vi "ELVIS III v1.1 Open UART.vi"(8 "error in (no error)":errorcluster, 10 "VISA resource name in":refnum<visa-resource-name>, 11 "Resource name":T1 caption="RIO Device") -> (0 "error out":errorcluster, 3 "VISA resource name":refnum<visa-resource-name>)   [LabVIEW 2021]
uses:
  <vilib>/userDefined/High Color/nirio_resource_hc.ctl
  <vilib>/myRIO/Common/Instrument Driver Framework/ELVIS III v1.0/UART/vis/ELVIS III v1.0 Build MUX Configuration UART.vi
  <vilib>/myRIO/Common/Instrument Driver Framework/ELVIS III v1.0/Resource Manager/vis/ELVIS III v1.0 Reserve Channel List.vi
  <vilib>/myRIO/Common/Instrument Driver Framework/ELVIS III v1.0/UART/vis/ELVIS III v1.0 Configure UART.vi
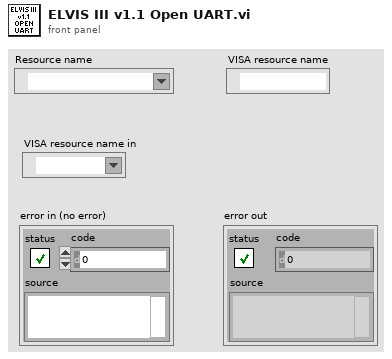
[diagram p1: front panel]
types:
  T1 = typedef "nirio_resource_hc.ctl" = tag
  T2 = typedef "Generic FPGA Reference.ctl" = refnum<k20>
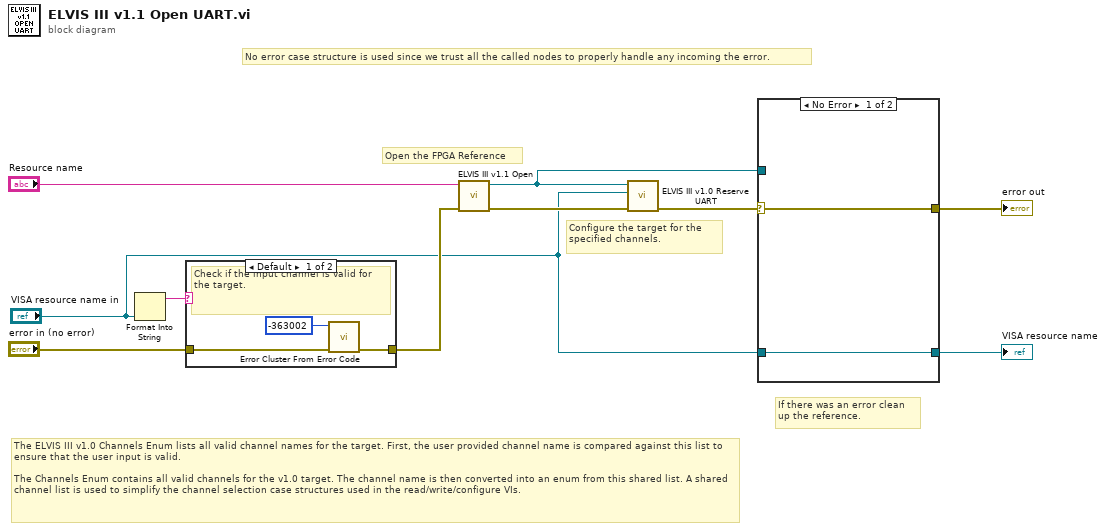
[diagram p0: block diagram]
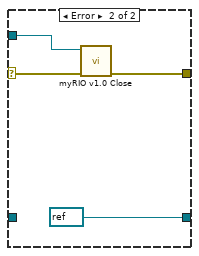
[diagram p3: hidden frame]
diagram:
  # "The ELVIS III v1.0 Channels Enum lists all valid channel names for the target. First, the user provided channel name is compared against this list to ensure that the user input is valid.\n\nThe Channels Enum contains all valid channels for the v1.0 target. The channel name is then converted into an enum from this shared list. A shared channel list is used to simplify the channel selection case structures used in the read/write/configure VIs."
  # "If there was an error clean up the reference."
  # "Configure the target for the specified channels."
  # "Open the FPGA Reference"
  # "No error case structure is used since we trust all the called nodes to properly handle any incoming the error."
  n1 = Format Into String("VISA resource name in") -> (resulting string=w5:string)  [unwired: 3 in, 1 out]
  n2 = case shown="Default" w5 {
    tunnel: "error in (no error)" -> [w12 w14]
    tunnel: [w11 w14] -> w3
    frame Default {
      # "Check if the input channel is valid for the target."
      n3 = call <vilib>:"Error Cluster From Error Code.vi"("error in (no error)"=w12, "error code (0)"=-363002) -> ("error out"=w11:errorcluster)  [unwired: 7 in]
    }
    frame "ASRL1::INSTR", "ASRL2::INSTR" {
      # "Check if the input channel is valid for the target."
    }
  }
  n4 = call <vilib>:"ELVIS III v1.1 Open.vi"("error in (no error)"=w3, "Resource name"="Resource name") -> ("error out"=w8:errorcluster, "myRIO FPGA Ref Out"=w6:T2)  [unwired: 8 in]
  n5 = call <vilib>:"ELVIS III v1.0 Reserve UART.vi"("error in (no error)"=w8, "VISA resource name in"="VISA resource name in", "myRIO FPGA Ref In"=w6) -> ("error out"=w7:errorcluster)  [unwired: 8 in]
  n6 = case shown="No Error" w7 {
    selector: w7 -> [w16 w20]
    tunnel: w6 -> [_ w18]
    tunnel: [w16 w19] -> w9
    tunnel: "VISA resource name in" -> [w15 _]
    tunnel: [w15 refnum<visa-resource-name> refnum ("VISA resource name in")] -> w1
    frame No Error {
    }
    frame Error {
      n7 = call <vilib>:"myRIO v1.0 Close.vi"("error in (no error)"=w20, "myRIO FPGA Ref In"=w18) -> ("error out"=w19:errorcluster)  [unwired: 9 in]
    }
  }
  "error out" <- w9
  "VISA resource name" <- w1
